vi "Print.vi"(8 "error in (no error)":errorcluster caption="错误输入（无错误）", 10 "text":string, 11 "path of image":path[](array[path])) -> (0 "error out":errorcluster caption="错误输出")   [LabVIEW 2019]
uses:
  <vilib>/Utility/NIReport.llb/Report Type.ctl
  <vilib>/Utility/NIReport.llb/Append Image to Report (path wrap).vi
  <vilib>/Utility/NIReport.llb/NI_report.lvclass
  <vilib>/Utility/NIReport.llb/NI_ReportGenerationCore.lvlib
  <vilib>/addons/_office/NI_ReportGenerationToolkit.lvlib
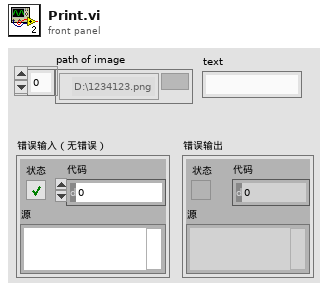
[diagram p1: front panel]
types:
  T1 = cluster{"top":dbl, "left":dbl, "right":dbl, "bottom":dbl}
  T2 = typedef "NI_ReportGenerationCore.lvlib/Report Type.ctl" = enum16{"HTML", "Word", "Excel"}
  T3 = enum16{"maximized", "minimized", "normal", "no change"}
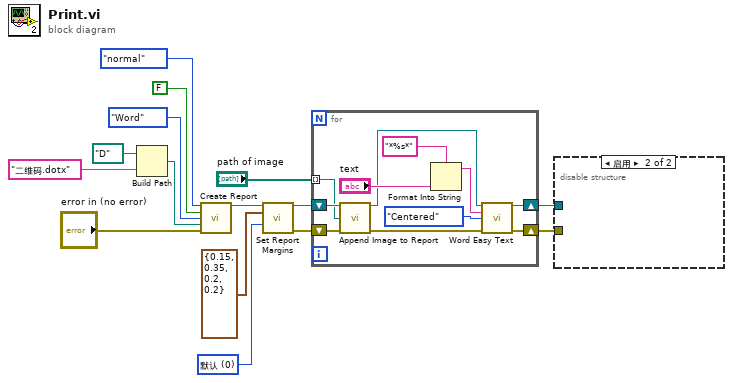
[diagram p0: block diagram]
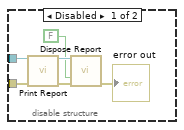
[diagram p2: hidden frame]
diagram:
  w10 = u16 0 items=["默认", "US", "公制"] ("measurement system (default)")
  n1 = Build Path(base path=path "D:/" ("基路径"), name or relative path="二维码.dotx") -> (appended path=w4:path)
  n2 = call <vilib>:"Create Report.vi"("window state (normal)"=T3."normal", "display alerts? (F)"=FALSE, "report type"=Report_Type."Word", "template (empty)"=w4, "error in (no error)"="error in (no error)") -> ("report out"=w12:refnum<class "NI_report.lvclass">)  [unwired: 9 in, 1 out]
  n3 = call-dynamic "Set Report Margins.vi"("report in"=w12, "margins (1.00)"=T1 {"top"=0.15, "left"=0.35, "right"=0.2, "bottom"=0.2}, "measurement system (default)"=w10) -> ("report out"=w2:refnum<class "NI_report.lvclass">, "error out"=w1:errorcluster)  [unwired: 10 in, 1 out]
  n4 = for {
    shift-right: [w19] -> w9
    shift-left: w2 -> [w26]
    shift-right: [w18] -> w8
    shift-left: w1 -> [w25]
    tunnel: "path of image" -> [w24] mode=indexing
    n5 = call-poly <vilib>:"Append Image to Report.vi"("report in"=w26, "path or URL of image"=w24, "error in (no error)"=w25) -> ("report out"=w17:refnum<class "NI_report.lvclass">, "error out"=w16:errorcluster)  [unwired: 9 in, 2 out]
    n6 = Format Into String(format string="*%s*" ("format string (%.3f)"), "text") -> (resulting string=w21:string)  [unwired: 2 in, 1 out]
    n7 = call <vilib>:"Word Easy Text.vi"("report in"=w17, "text"=w21, "alignment (left)"=enum16{"Left", "Centered", "Right", "Justify"}."Centered", "error in (no error)"=w16) -> ("report out"=w19:refnum<class "NI_report.lvclass">, "error out"=w18:errorcluster)  [unwired: 9 in, 1 out]
  }
  n8 = disable-structure shown="启用" {
    disable-tunnel: w9 -> [w32 _]
    disable-tunnel: w8 -> [w31 _]
    frame Disabled {
      n9 = call-dynamic "Print Report.vi"("report in"=w32, "error in (no error)"=w31) -> ("report out"=w30:refnum<class "NI_report.lvclass">, "error out"=w29:errorcluster)  [unwired: 12 in]
      n10 = call-dynamic "Dispose Report.vi"("report in"=w30, "save changes? (F)"=FALSE, "error in (no error)"=w29) -> ("error out"=→"error out":errorcluster)  [unwired: 12 in]
    }
    frame Enabled {
    }
  }
